vi "Generate_WF_Regression_Dataset.vi"(8 "error in (no error)":errorcluster) -> (0 "error out":errorcluster, 3 "DataSets_All(In1D_Out1D)":T1)   [LabVIEW 2020]
uses:
  <vilib>/Ngene/DeepLTK/Toolkit/NN_Data/API/DataSet_Types/NN_DataSets_All(In1D_Out1D).ctl
  <vilib>/Ngene/DeepLTK/Toolkit/NN_Data/API/DataSet_Types/NN_DataSet(In1D_Out1D).ctl
  <vilib>/Ngene/DeepLTK/Toolkit/NN_Data/API/DataRef_Types/NN_Data_ref(2D_SGL).ctl
  <vilib>/Ngene/DeepLTK/Toolkit/NN_Data/API/DataRef_Types/NN_Data_ref(1D_I32).ctl
  <vilib>/Ngene/DeepLTK/Toolkit/Deep_Learning_Toolkit_by_Ngene.lvlib
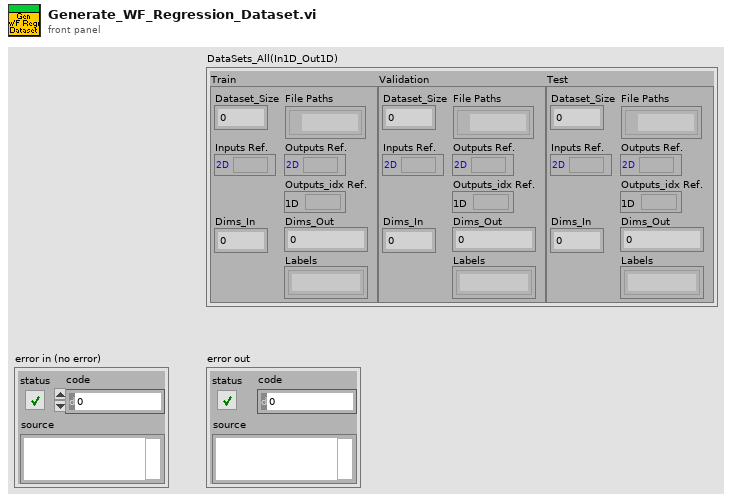
[diagram p1: front panel]
types:
  T1 = typedef "Deep_Learning_Toolkit_by_Ngene.lvlib/NN_DataSets_All(In1D_Out1D).ctl" = cluster{"Train":T2, "Validation":T2, "Test":T2}
  T2 = typedef "Deep_Learning_Toolkit_by_Ngene.lvlib/NN_DataSet(In1D_Out1D).ctl" = cluster{"Inputs Ref.":T3, "Outputs Ref.":T3, "Dims_In":i32, "Dataset_Size":i32, "Outputs_idx Ref.":T4, "Dims_Out":i32, "Labels":string[], "File Paths":path[]}
  T3 = typedef "Deep_Learning_Toolkit_by_Ngene.lvlib/NN_Data_ref(2D_SGL).ctl" = refnum<data-value>
  T4 = typedef "Deep_Learning_Toolkit_by_Ngene.lvlib/NN_Data_ref(1D_I32).ctl" = refnum<data-value>
  T5 = enum16{"Sine Wave", "Triangle Wave", "Square Wave", "Sawtooth Wave", "Noise"}[]
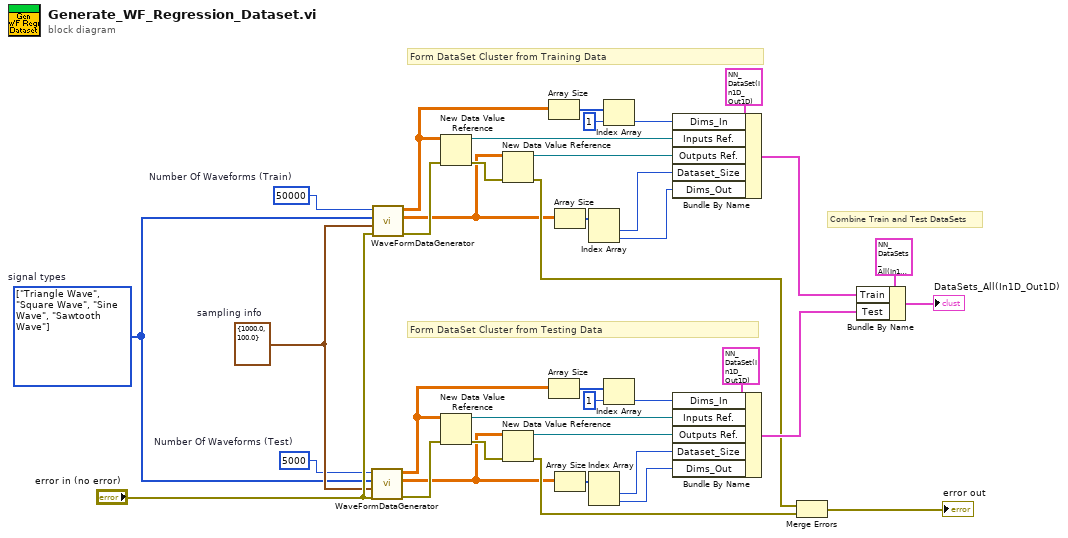
[diagram p0: block diagram]
diagram:
  w30 = 5000  # Number Of Waveforms (Test)
  w36 = cluster{"Fs":dbl, "#s":dbl} {"Fs"=1000.0, "#s"=100.0}  # sampling info
  w17 = 50000  # Number Of Waveforms (Train)
  w10 = T5 [enum."Triangle Wave", enum."Square Wave", enum."Sine Wave", enum."Sawtooth Wave"] items=["Sine Wave", "Triangle Wave", "Square Wave", "Sawtooth Wave", "Noise"]  # signal types
  # "Combine Train and Test DataSets"
  # "Form DataSet Cluster from Testing Data"
  # "Form DataSet Cluster from Training Data"
  n1 = call "WaveFormDataGenerator.vi"("error in"="error in (no error)", "sampling info"=w36, "Signal Types/Classes"=w10, "Number of Waveforms per Signal Type"=w30) -> ("error out"=w31:errorcluster, "Proparties"=w6:sgl[][], "Generated Waveform"=w28:sgl[][])  [unwired: 5 in]
  n2 = call "WaveFormDataGenerator.vi"("error in"="error in (no error)", "sampling info"=w36, "Signal Types/Classes"=w10, "Number of Waveforms per Signal Type"=w17) -> ("error out"=w16:errorcluster, "Proparties"=w9:sgl[][], "Generated Waveform"=w20:sgl[][])  [unwired: 5 in]
  n3 = New Data Value Reference(data value=w20, error in=w16) -> (data value reference=w19:refnum<data-value>, error out=w11:errorcluster)
  n4 = New Data Value Reference(data value=w28, error in=w31) -> (data value reference=w29:refnum<data-value>, error out=w34:errorcluster)
  n5 = New Data Value Reference(data value=w9, error in=w11) -> (data value reference=w18:refnum<data-value>, error out=w15:errorcluster)
  n6 = New Data Value Reference(data value=w6, error in=w34) -> (data value reference=w5:refnum<data-value>, error out=w32:errorcluster)
  n7 = Array Size(array=w20) -> (size(s)=w21:i32[])
  n8 = Array Size(array=w28) -> (size(s)=w27:i32[])
  n9 = Array Size(array=w9) -> (size(s)=w22:i32[])
  n10 = Array Size(array=w6) -> (size(s)=w26:i32[])
  n11 = Index Array(array=w22) -> (element #1=w4:i32, element #2=w3:i32)  [unwired: 2 in]
  n12 = Index Array(array=w26) -> (element #1=w2:i32, element #2=w1:i32)  [unwired: 2 in]
  n13 = Index Array(array=w21, index=1) -> (element=w7:i32)
  n14 = Index Array(array=w27, index=1) -> (element=w8:i32)
  n15 = Bundle By Name(cluster=T2 {"Inputs Ref."=refnum, "Outputs Ref."=refnum, "Dims_In"=0, "Dataset_Size"=0, "Outputs_idx Ref."=refnum, "Dims_Out"=0, "Labels"=[], "File Paths"=[]} ("Dataset(In1D_Out1D)"), "Dims_In"=w7, "Inputs Ref."=w19, "Outputs Ref."=w18, "Dataset_Size"=w4, "Dims_Out"=w3) -> (w14:T2)
  n16 = Bundle By Name(cluster=T2 {"Inputs Ref."=refnum, "Outputs Ref."=refnum, "Dims_In"=0, "Dataset_Size"=0, "Outputs_idx Ref."=refnum, "Dims_Out"=0, "Labels"=[], "File Paths"=[]} ("Dataset(In1D_Out1D)"), "Dims_In"=w8, "Inputs Ref."=w29, "Outputs Ref."=w5, "Dataset_Size"=w2, "Dims_Out"=w1) -> (w35:T2)
  n17 = Merge Errors(w15, w32) -> (→"error out":errorcluster)
  n18 = Bundle By Name(cluster=T1 {"Train"={"Inputs Ref."=refnum, "Outputs Ref."=refnum, "Dims_In"=0, "Dataset_Size"=0, "Outputs_idx Ref."=refnum, "Dims_Out"=0, "Labels"=[], "File Paths"=[]}, "Validation"={"Inputs Ref."=refnum, "Outputs Ref."=refnum, "Dims_In"=0, "Dataset_Size"=0, "Outputs_idx Ref."=refnum, "Dims_Out"=0, "Labels"=[], "File Paths"=[]}, "Test"={"Inputs Ref."=refnum, "Outputs Ref."=refnum, "Dims_In"=0, "Dataset_Size"=0, "Outputs_idx Ref."=refnum, "Dims_Out"=0, "Labels"=[], "File Paths"=[]}} ("DataSets_All(In1D_Out1D)"), "Train"=w14, "Test"=w35) -> (→"DataSets_All(In1D_Out1D)":T1)
